vi "Sea battle.vi"() -> ()   [LabVIEW 2012]
doc: "Sends a specified waveform through a TCP port. The VI first listens for a connection and, once established, sends the number of bytes to be sent followed by the data. After the data is sent, the VI waits for an 'all received' signal from the client and then breaks the connection.\n\n<B>Note:</B> Requires the Data Client.vi located in the same library as this VI."
panel:
  in  "А        Б       В        Г      Д   2":bool[][](array[boolean]) caption="А        Б       В        Г      Д       Е"
  in  "А        Б       В        Г      Д":bool[][](array[boolean])
  in  "Прийом даних":bool
  in  "Port 2":u16=6340 min=1025 step=1
  in  "IP суперника":string="localhost"
  in  "Передача даних":bool
  in  "Припинити гру":bool
  in  "Port 1":u16=6340 min=1025 step=1
  # "А       Б       В       Г       Д"
  # "А       Б       В       Г       Д"
  # "0\n\n1\n\n2\n\n3\n\n4"
  # "0\n\n1\n\n2\n\n3\n\n4"
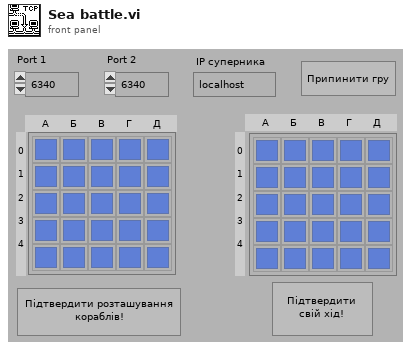
[diagram p1: front panel]
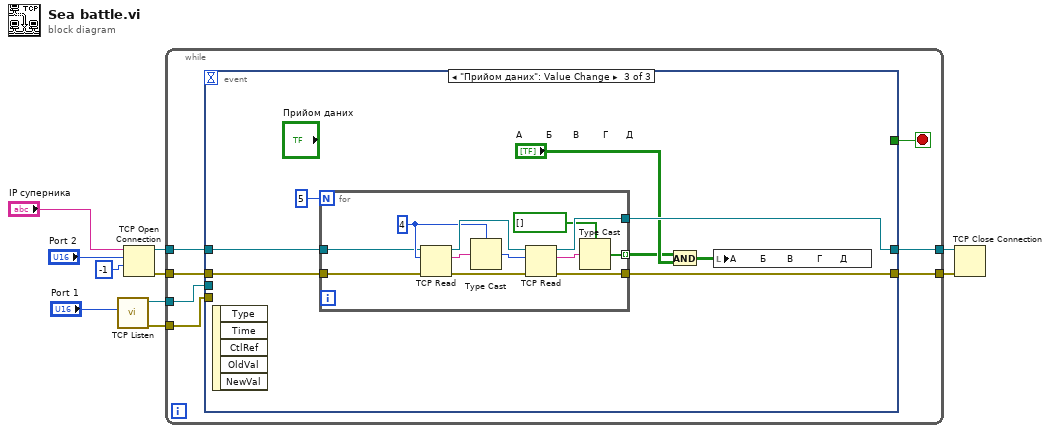
[diagram p0: block diagram]
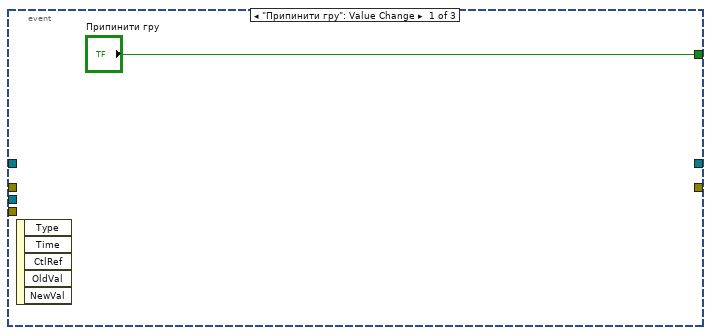
[diagram p2: hidden frame]
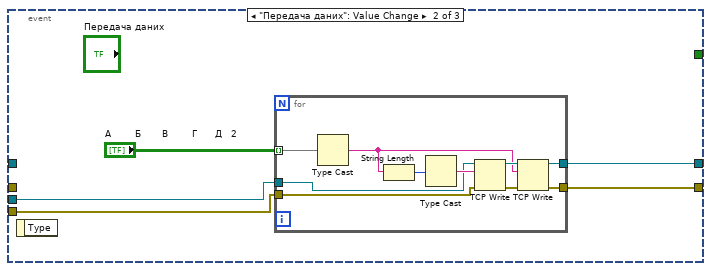
[diagram p3: hidden frame]
diagram:
  n1 = call <vilib>:"TCP Listen.vi"("port"="Port 1") -> ("error out"=w9:errorcluster, "connection ID"=w10:refnum<k5>)  [unwired: 6 in, 3 out]
  n2 = TCP Open Connection(address="IP суперника", remote port or service name="Port 2", timeout ms (60000)=-1) -> (connection ID=w4:refnum<k5>, error out=w3:errorcluster)  [unwired: 1 in, 1 out]
  n3 = while {
    tunnel: w10 -> [w16]
    tunnel: w9 -> [w15]
    tunnel: [w14] -> w8
    tunnel: [w13] -> w7
    tunnel: w4 -> [w12]
    tunnel: w3 -> [w11]
    stop <- w17 stop-if-true
    n4 = event shown="[2] \"Прийом даних\": Value Change" {
      selector: _ -> [_ _ _]
      dyn-events: _ -> [_ _ _]
      timeout: _ -> [_ _ _]
      tunnel: ["Припинити гру" _ _] -> w17
      tunnel: w16 -> [_ w23 _]
      tunnel: w15 -> [_ w22 _]
      tunnel: [_ w21 w41] -> w14
      tunnel: [_ w20 w40] -> w13
      tunnel: w12 -> [_ _ w37]
      tunnel: w11 -> [_ _ w39]
      event "Припинити гру": Value Change {
        n5 = event-data() -> ()  [unwired: 1 in, 5 out]
      }
      event "Передача даних": Value Change {
        n6 = event-data() -> ()  [unwired: 1 in, 1 out]
        n7 = for {
          tunnel: w23 -> [w28]
          tunnel: w22 -> [w27]
          tunnel: [w26] -> w21
          tunnel: [w25] -> w20
          tunnel: "А        Б       В        Г      Д   2" -> [w24] mode=indexing
          n8 = Type Cast(x=w24) -> (*(type *) &x=w29:string)  [unwired: 1 in]
          n9 = String Length(string=w29) -> (length=w31:i32)
          n10 = Type Cast(x=w31) -> (*(type *) &x=w30:string)  [unwired: 1 in]
          n11 = TCP Write(connection ID=w28, data in=w30, error in (no error)=w27) -> (connection ID out=w32:refnum<k5>, error out=w33:errorcluster)  [unwired: 1 in, 1 out]
          n12 = TCP Write(connection ID=w32, data in=w29, error in (no error)=w33) -> (connection ID out=w26:refnum<k5>, error out=w25:errorcluster)  [unwired: 1 in, 1 out]
        }
      }
      event "Прийом даних": Value Change {
        n13 = event-data() -> ()  [unwired: 1 in, 5 out]
        n14 = for {
          N: 5 -> [_]
          tunnel: [w47] -> w41
          tunnel: [w46] -> w40
          tunnel: w37 -> [w45]
          tunnel: w39 -> [w44]
          tunnel: [w42] -> w34 mode=indexing
          w49 = 4
          n15 = TCP Read(connection ID=w45, bytes to read=w49, error in (no error)=w44) -> (connection ID out=w53:refnum<k5>, data out=w48:string, error out=w50:errorcluster)  [unwired: 2 out]
          n16 = Type Cast(type=w49, x=w48) -> (*(type *) &x=w51:i32)
          n17 = TCP Read(connection ID=w53, bytes to read=w51, error in (no error)=w50) -> (connection ID out=w47:refnum<k5>, data out=w52:string, error out=w46:errorcluster)  [unwired: 2 out]
          n18 = Type Cast(type=bool[] [], x=w52) -> (*(type *) &x=w42:bool[])
        }
        n19 = And(x=w34, y="А        Б       В        Г      Д") -> (x .and. y?=w35:bool[][])
        n20 = local write "А        Б       В        Г      Д"(w35) -> ()
      }
    }
  }
  n21 = TCP Close Connection(connection ID=w8, error in (no error)=w7) -> ()  [unwired: 1 in, 2 out]
